vi "Paskevits_Vladislav_Capfit.vi"() -> ()   [LabVIEW 2018]
doc: "This Sub-Vi should display three lines on the same graph - the calculated curve, the calculated curve with the added noise, and the loading or discharging graph corresponding to the best approximation parameters depending on the Charging value of the input (approximate curve)."
uses:
  <vilib>/Analysis/NI_AALBase.lvlib
panel:
  out "Waveform Graph":cluster{dbl, "Ajasamm ( 0.01 sec)":dbl, dbl[]}[](graph)
  out "Discharging Non-linear coefficients 2":dbl
  out "Discharging Best Fit 2":dbl
  out "Charging Non-linear coefficients":dbl
  out "Charging Best Fit":dbl
  in  "stop":bool
  in  "amplitude":dbl=1.0 format="%0.2f"
  in  "amplitude 2":dbl=1.0 format="%0.2f"
  out "Charging output waveform":waveform(dbl)
  out "DIsharging output waveform 2":waveform(dbl)
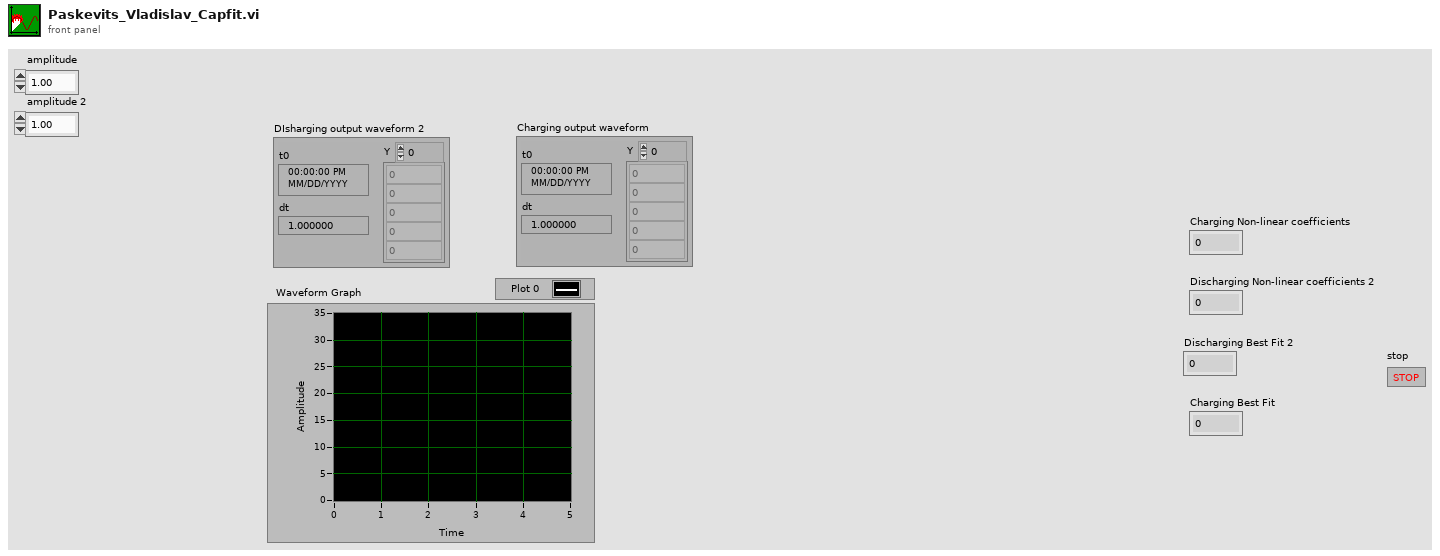
[diagram p1: front panel]
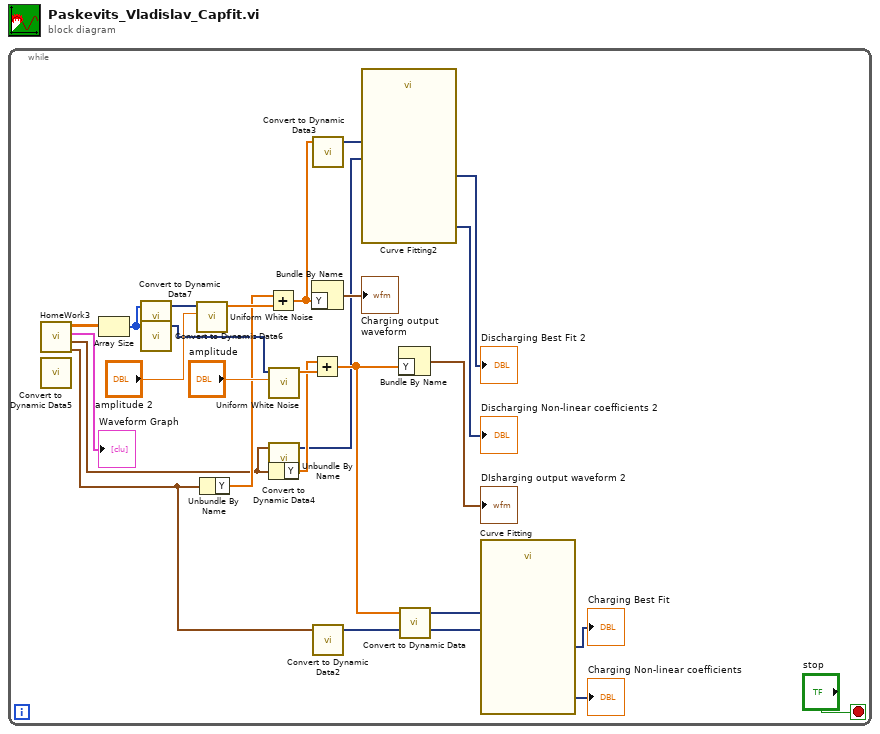
[diagram p0: block diagram]
diagram:
  n1 = while {
    stop <- "stop" stop-if-true
    n2 = call "HomeWork3.vi"() -> ("Time array"=w7:dbl[][], "Waveform Graph"=→"Waveform Graph":cluster{dbl, "Ajasamm ( 0.01 sec)":dbl, dbl[]}[], "Discharging waveform"=w6:waveform(dbl), "Charging waveform"=w2:waveform(dbl))  [unwired: 7 in]
    n3 = call "Convert to Dynamic Data5"() -> ()  [unwired: 4 in, 1 out]
    n4 = Array Size(array=w7) -> (size(s)=w3:i32[])
    n5 = call "Convert to Dynamic Data7"("Array"=w3) -> ("Dynamic Data Type"=w4:dynamicdata)  [unwired: 3 in]
    n6 = call "Convert to Dynamic Data6"("Array"=w3) -> ("Dynamic Data Type"=w5:dynamicdata)  [unwired: 3 in]
    n7 = call <vilib>:"Uniform White Noise.vi"("amplitude"="amplitude 2", "samples"=w4) -> ("uniform white noise"=w21:dbl[])  [unwired: 8 in, 1 out]
    n8 = Unbundle By Name(w2) -> ("Y"=w20:dbl[])
    n9 = Add(x=w20, y=w21) -> (x+y=w14:dbl[])
    n10 = call <vilib>:"Uniform White Noise.vi"("amplitude"="amplitude", "samples"=w5) -> ("uniform white noise"=w24:dbl[])  [unwired: 8 in, 1 out]
    n11 = call "Convert to Dynamic Data4"("Array"=w6) -> ("Dynamic Data Type"=w12:dynamicdata)  [unwired: 3 in]
    n12 = Unbundle By Name(w6) -> ("Y"=w23:dbl[])
    n13 = Bundle By Name("Y"=w14) -> (→"Charging output waveform":waveform(dbl))  [unwired: 1 in]
    n14 = Add(x=w23, y=w24) -> (x+y=w17:dbl[])
    n15 = call "Convert to Dynamic Data3"("Array"=w14) -> ("Dynamic Data Type"=w13:dynamicdata)  [unwired: 3 in]
    n16 = call "Convert to Dynamic Data2"("Array"=w2) -> ("Dynamic Data Type"=w15:dynamicdata)  [unwired: 3 in]
    n17 = call "Curve Fitting2"("Locations"=w12, "Signals"=w13) -> ("best fit"=→"Discharging Best Fit 2":dynamicdata, "non-linear coefficients"=→"Discharging Non-linear coefficients 2":dynamicdata)  [unwired: 5 in, 3 out]
    n18 = Bundle By Name("Y"=w17) -> (→"DIsharging output waveform 2":waveform(dbl))  [unwired: 1 in]
    n19 = call "Convert to Dynamic Data"("Array"=w17) -> ("Dynamic Data Type"=w16:dynamicdata)  [unwired: 3 in]
    n20 = call "Curve Fitting"("Locations"=w15, "Signals"=w16) -> ("best fit"=→"Charging Best Fit":dynamicdata, "non-linear coefficients"=→"Charging Non-linear coefficients":dynamicdata)  [unwired: 5 in, 3 out]
  }
